vi "Configure Device.vi"(8 "error in":errorcluster, 11 "DAQ Device in":refnum<class "DAQ Device.lvclass">) -> (0 "error out":errorcluster, 3 "DAQ Device out":refnum<class "DAQ Device.lvclass">)   [LabVIEW 2014, in "DAQ Device.lvclass"]
doc: "Get information from theh configuration session to configure the device for operation. The default is to do nothing."
uses:
  DAQ Device.lvclass
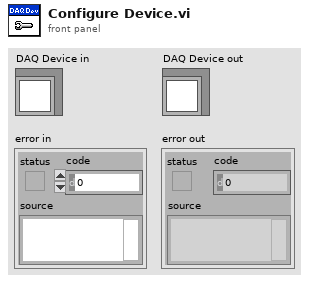
[diagram p1: front panel]
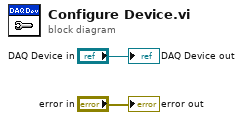
[diagram p0: block diagram]
diagram:
  "error out" <- "error in"
  "DAQ Device out" <- "DAQ Device in"
